vi "CheckForAlreadyRegistered.vi"(1 "ROS":T1, 2 "Registered":T1[](array[typedef])) -> (0 "index of element":i32)   [LabVIEW 2015]
doc: "Compares ROS definitions to prevent duplicates"
uses:
  _ROSControl.ctl
  _ROSDirection.ctl
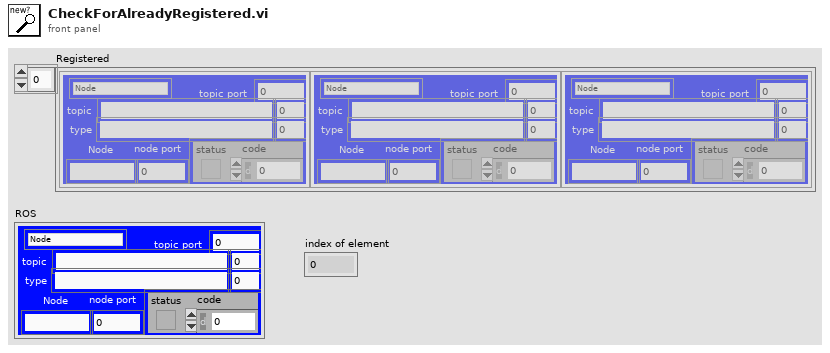
[diagram p1: front panel]
types:
  T1 = typedef "_ROSControl.ctl" = cluster{"topic port":u16, "Node":string, "topic":string, "type":string, "node port":u16, "error ":errorcluster, "Direction":T2, "Update (ms)":u16, "FIFO size":u16}
  T2 = typedef "_ROSDirection.ctl" = enum16{"Node", "Publisher", "Subscriber", "ServiceClient", "ServiceProvider"}
  T3 = cluster{"Node":string, "topic":string, "Direction":T2}
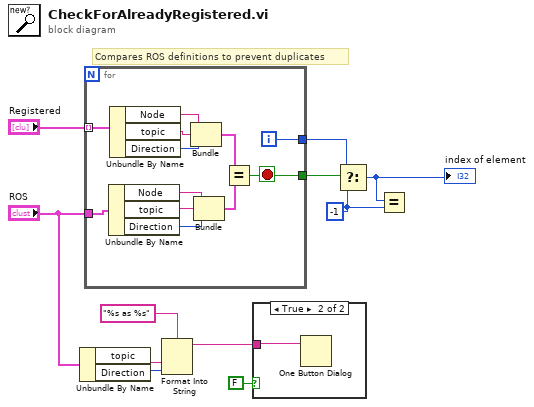
[diagram p0: block diagram]
diagram:
  w7 = -1 ("f")
  # "Compares ROS definitions to prevent duplicates"
  n1 = Unbundle By Name("ROS") -> ("topic"=w2:string, "Direction"=w5:T2)
  n2 = for {
    tunnel: "Registered" -> [w23] mode=indexing
    tunnel: "ROS" -> [w22]
    tunnel: [w13] -> w10
    tunnel: [w12] -> w9
    i -> [w12]
    stop <- w13 stop-if-true
    n3 = Unbundle By Name(w22) -> ("Node"=w17:string, "topic"=w18:string, "Direction"=w16:T2)
    n4 = Unbundle By Name(w23) -> ("Node"=w21:string, "topic"=w20:string, "Direction"=w19:T2)
    n5 = Bundle("Node"=w21, "topic"=w20, "Direction"=w19) -> (w15:T3)  [unwired: 1 in]
    n6 = Bundle("Node"=w17, "topic"=w18, "Direction"=w16) -> (w14:T3)  [unwired: 1 in]
    n7 = Equal?(x=w15, y=w14) -> (x = y?=w13:bool)
  }
  n8 = Format Into String(format string="%s as %s", w2, w5) -> (resulting string=w3:string)  [unwired: 2 in, 1 out]
  n9 = case shown="True" FALSE {
    tunnel: w3 -> [_ w24]
    frame False {
    }
    frame True {
      n10 = One Button Dialog(message=w24) -> ()  [unwired: 1 in, 1 out]
    }
  }
  n11 = Select(t=w9, s=w10, f=w7) -> (s? t:f=w8:i32)
  "index of element" <- w8
  n12 = Equal?(x=w8, y=w7) -> ()  [unwired: 1 out]
